vi "PTSequencer.execute step.vi"(0 "i ref in":refnum<vi>, 3 "ms timeout (10000)":i32=10000, 5 "error in (no error)":errorcluster) -> (14 "i ref out":refnum<vi>, 16 "next step":string, 17 "timed out":bool, 19 "error out":errorcluster)   [LabVIEW 2014, in "PTSequencer.lvlib"]
uses:
  PTSequencer.lvlib
  CS_Core/BaseProcess/BaseProcess.lvlib
  CS_Core/CSSystem/CSSystemLib/CSSystemLib.lvlib
  CS_Core/BaseSM/BaseSM.lvlib
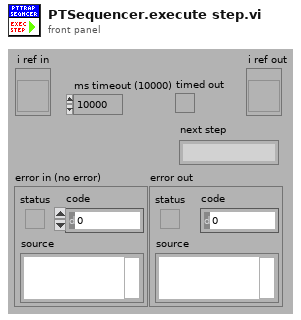
[diagram p1: front panel]
types:
  T1 = typedef "PTSequencer.lvlib/PTSequencer.i attribute.ctl" = cluster{"subsequence":bool, "mode":T2, "i step":i32, "nofLoops":i32, "i loop":i32, "Running":bool, "Paused":bool, "step done":bool, "loop done":bool, "seq done":bool, "DIM IDs":cluster{"step done":i32, "loop done":i32, "seq done":i32, "i step":i32, "i loop":i32}, "use stop conditions":bool, "stop conditions":T3[], "Step List":T5[], "DIM subsriptions":string[], "stop cond indexes":i32[], "step cond indexes":cluster{"step condition IDs":cluster{"step ID":i32, "condition ID":i32}[]}[], "Delay Start Time":timestamp, "status":string, "stopping":bool}
  T2 = typedef "PTSequencer.lvlib/PTSequencer.mode.ctl" = enum16{"single", "loop", "for loop"}
  T3 = typedef "PTSequencer.lvlib/PTSequencer.DIM service condition.ctl" = cluster{"DIM service":string, "descr":string, "nomValue":T4, "actValue":T4, "matched":bool, "DIM Status":cluster{"no link":bool, "quality":i32, "Time Stamp":timestamp}}
  T4 = typedef "CoreDefs.rawDataType.ctl" = i8[]
  T5 = typedef "PTSequencer.lvlib/PTSequencer.step.ctl" = cluster{"description":string, "object parameters":cluster{"object":string, "selector":string, "descriptor":string, "data":T4, "subsequence":bool, "call mode":enum16{"Simple DIM", "Synchronous"}, "data in":T4}, "result action":cluster{"check":bool, "passed":enum16{"Next", "Previous", "Repeat", "Jump"}, "failed":enum16{"Next", "Previous", "Repeat", "Jump"}, "jumpID_passed":i32, "jumpID_failed":i32}, "conditions":T3[], "fulfilled ":bool, "use delay":bool, "delay time (s)":dbl, "ID":i32}
  T6 = typedef "CoreDefs.call_type.ctl" = cluster{"Object":string, "Selector":string, "CallType":enum16{"simple", "synchronous", "asynchronous"}, "Async Object":string, "Async Selector":string, "Data Descriptor":T7, "Data":T4, "Error #":i32, "Expire":u32}
  T7 = typedef "BaseProcess.lvlib/BaseProcess.descriptor string definition.ctl" = string
  T8 = typedef "BaseSM.lvlib/BaseSM.i attribute.ctl" = cluster{"stateError":i32, "stateStatus":string, "stateQuality":T9, "ProcStateRef":refnum<vi>, "thread ref":refnum<vi>, "actState":string, "reqState":string, "SMQueue":refnum<queue>, "stateErrorID":i32, "stateStatusID":i32}
  T9 = typedef "BaseSM.lvlib/BaseSM.stateQuality.ctl" = i16
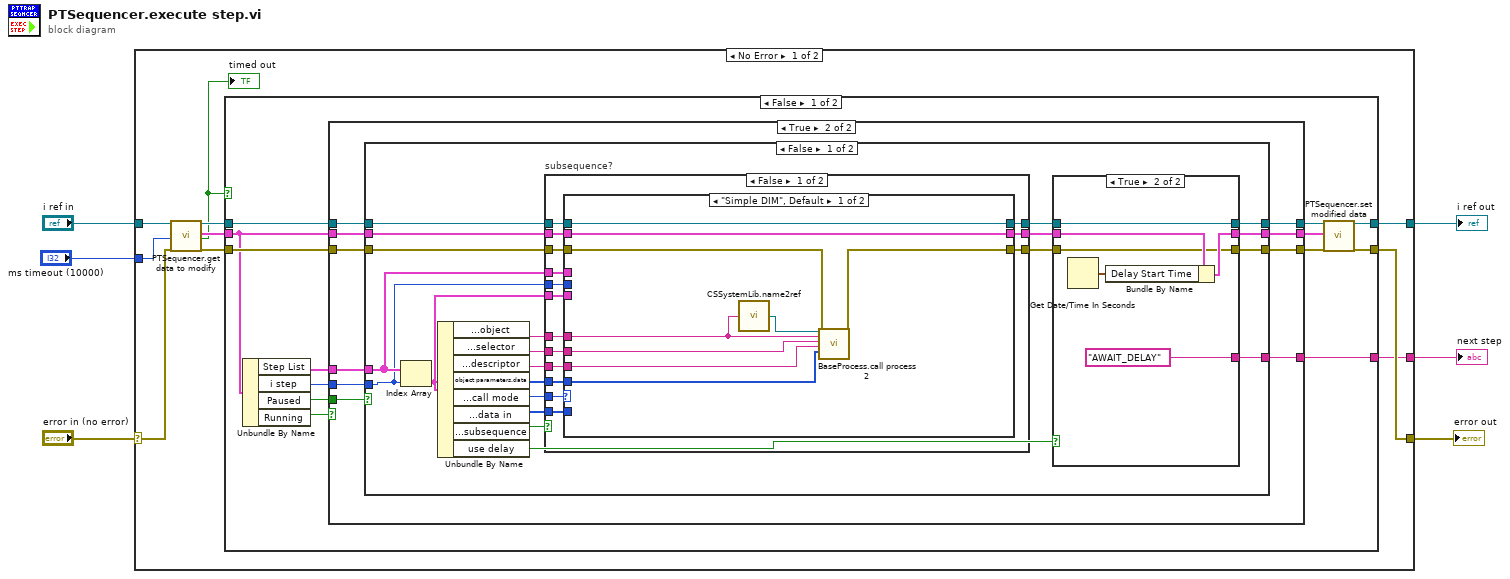
[diagram p0: block diagram]
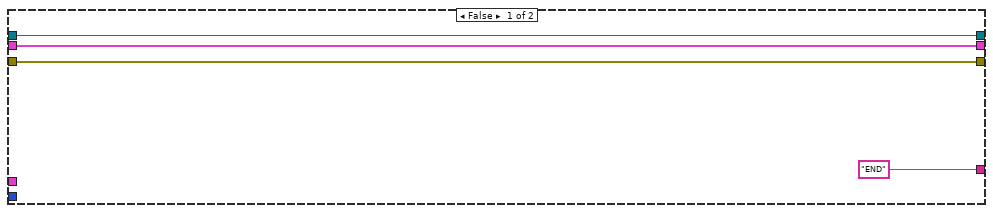
[diagram p2: hidden frame]
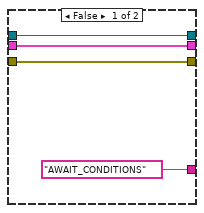
[diagram p3: hidden frame]
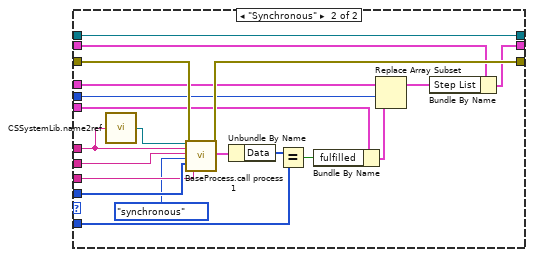
[diagram p4: hidden frame]
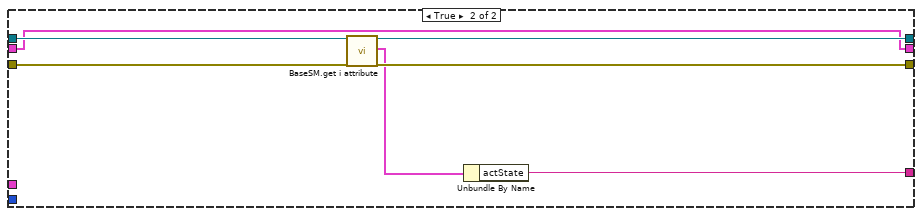
[diagram p6: hidden frame]
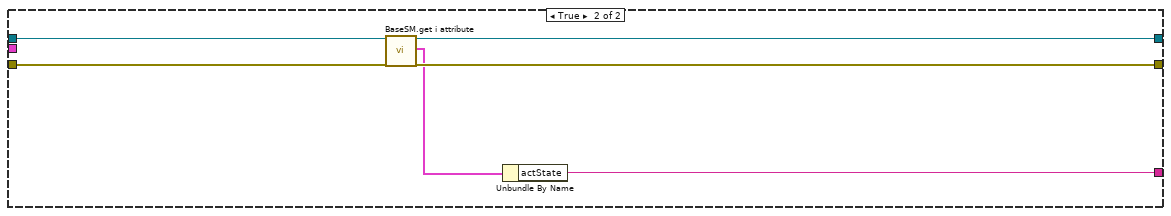
[diagram p7: hidden frame]
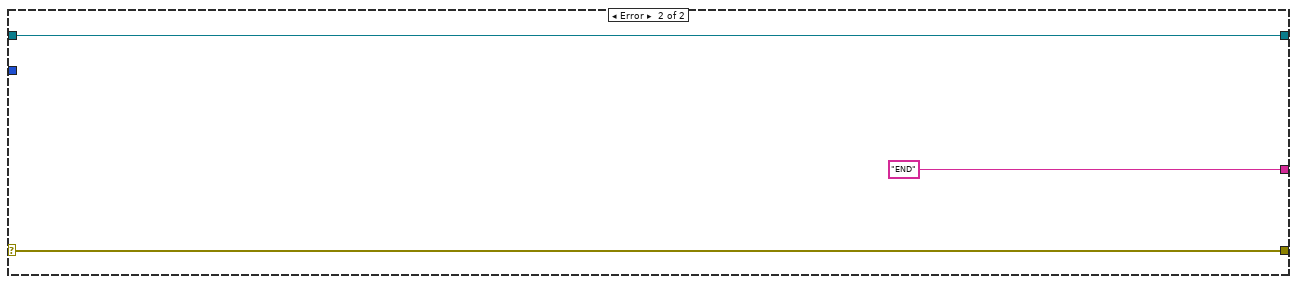
[diagram p8: hidden frame]
diagram:
  n1 = case shown="No Error" "error in (no error)" {
    selector: "error in (no error)" -> [w12 w136]
    tunnel: "i ref in" -> [w16 w137]
    tunnel: [w10 w136] -> w5
    tunnel: [w11 w137] -> w4
    tunnel: "ms timeout (10000)" -> [w8 _]
    tunnel: [w7 "END"] -> w1
    frame No Error {
      n2 = call "PTSequencer.get data to modify.vi"("i ref in"=w16, "ms timeout (10000)"=w8, "error in (no error)"=w12) -> ("i ref out"=w13:refnum<vi>, "i attribute"=w15:T1, "timed out"=w9:bool, "error out"=w14:errorcluster)  [unwired: 13 in]
      "timed out" <- w9
      n3 = case shown="False" w9 {
        tunnel: w15 -> [w23 _]
        tunnel: w14 -> [w29 w133]
        tunnel: w13 -> [w28 w134]
        tunnel: [w27 w132] -> w11
        tunnel: [w25 w131] -> w10
        tunnel: [w19 w129] -> w7
        frame False {
          n4 = Unbundle By Name(w23) -> ("Step List"=w22:T5[], "i step"=w21:i32, "Paused"=w17:bool, "Running"=w18:bool)
          n5 = case shown="True" w18 {
            tunnel: w29 -> [w30 w43]
            tunnel: w28 -> [w32 w42]
            tunnel: [w32 w41] -> w26
            tunnel: [w30 w40] -> w24
            tunnel: w23 -> [w31 w39]
            tunnel: w22 -> [_ w38]
            tunnel: w21 -> [_ w37]
            tunnel: [w31 w36] -> w20
            tunnel: ["END" w35] -> w19
            tunnel: w17 -> [_ w34]
            frame False {
            }
            frame True {
              n6 = case shown="False" w34 {
                tunnel: w43 -> [w63 w127]
                tunnel: w42 -> [w62 w128]
                tunnel: [w46 w126] -> w41
                tunnel: [w44 w125] -> w40
                tunnel: w39 -> [w57 w122]
                tunnel: w38 -> [w54 _]
                tunnel: w37 -> [w53 _]
                tunnel: [w49 w122] -> w36
                tunnel: [w48 w123] -> w35
                frame False {
                  n7 = Index Array(array=w54, index=w53) -> (element=w52:T5)
                  n8 = Unbundle By Name(w52) -> ("object parameters.object"=w61:string, "object parameters.selector"=w60:string, "object parameters.descriptor"=w59:string, "object parameters.data"=w58:T4, "object parameters.call mode"=w56:enum16{"Simple DIM", "Synchronous"}, "object parameters.data in"=w55:T4, "object parameters.subsequence"=w64:bool, "use delay"=w51:bool)
                  n9 = case "subsequence?" shown="False" w64 {
                    tunnel: w63 -> [w85 w119]
                    tunnel: w62 -> [w80 w121]
                    tunnel: w61 -> [w89 _]
                    tunnel: w60 -> [w88 _]
                    tunnel: w59 -> [w87 _]
                    tunnel: w58 -> [w86 _]
                    tunnel: [w79 w121] -> w47
                    tunnel: [w84 w119] -> w45
                    tunnel: [w78 w120] -> w50
                    tunnel: w57 -> [w81 w120]
                    tunnel: w56 -> [w83 _]
                    tunnel: w55 -> [w82 _]
                    tunnel: w54 -> [w77 _]
                    tunnel: w53 -> [w76 _]
                    tunnel: w52 -> [w75 _]
                    frame False {
                      n10 = case shown="\"Simple DIM\", Default" w83 {
                        tunnel: w89 -> [w97 w117]
                        tunnel: w88 -> [w96 w116]
                        tunnel: w87 -> [w95 w112]
                        tunnel: w86 -> [w90 w115]
                        tunnel: w85 -> [w94 w114]
                        tunnel: [w93 w113] -> w84
                        tunnel: w82 -> [_ w108]
                        tunnel: w81 -> [w91 w107]
                        tunnel: w80 -> [w92 w102]
                        tunnel: [w92 w102] -> w79
                        tunnel: [w91 w103] -> w78
                        tunnel: w77 -> [_ w106]
                        tunnel: w76 -> [_ w104]
                        tunnel: w75 -> [_ w101]
                        frame "Simple DIM", Default {
                          n11 = call "CSSystemLib.name2ref.vi"("name"=w97) -> ("obj refnum"=w98:refnum<vi>)
                          n12 = call "BaseProcess.call process 2.vi"("i ref in"=w98, "Object"=w97, "Selector"=w96, "Data Descriptor"=w95, "Data"=w90, "error in (no error)"=w94) -> ("error out"=w93:errorcluster)  [unwired: 12 in, 1 out]
                        }
                        frame "Synchronous" {
                          n13 = call "CSSystemLib.name2ref.vi"("name"=w117) -> ("obj refnum"=w118:refnum<vi>)
                          n14 = call "BaseProcess.call process 1.vi"("i ref in"=w118, "Object"=w117, "Selector"=w116, "CallType"=enum16{"simple", "synchronous", "asynchronous"}."synchronous", "Data"=w115, "error in (no error)"=w114, "Data Descriptor"=w112) -> ("call cluster out"=w110:T6, "error out"=w113:errorcluster)  [unwired: 10 in, 1 out]
                          n15 = Unbundle By Name(w110) -> ("Data"=w109:T4)
                          n16 = Equal?(x=w109, y=w108) -> (x = y?=w100:bool)
                          n17 = Bundle By Name(cluster=w101, "fulfilled"=w100) -> (w99:T5)
                          n18 = Replace Array Subset(array=w106, new element=w99, index=w104) -> (w105:T5[])
                          n19 = Bundle By Name(cluster=w107, "Step List"=w105) -> (w103:T1)
                        }
                      }
                    }
                    frame True {
                    }
                  }
                  n20 = case shown="True" w51 {
                    tunnel: w50 -> [w68 w74]
                    tunnel: [w68 w72] -> w49
                    tunnel: ["AWAIT_CONDITIONS" "AWAIT_DELAY"] -> w48
                    tunnel: w47 -> [w66 w70]
                    tunnel: [w66 w70] -> w46
                    tunnel: w45 -> [w65 w69]
                    tunnel: [w65 w69] -> w44
                    frame False {
                    }
                    frame True {
                      n21 = Get Date/Time In Seconds() -> (seconds since 1Jan1904=w73:timestamp)
                      n22 = Bundle By Name(cluster=w74, "Delay Start Time"=w73) -> (w72:T1)
                    }
                  }
                }
                frame True {
                  n23 = call "BaseSM.get i attribute.vi"("i ref in"=w128, "error in (no error)"=w127) -> ("i ref out"=w126:refnum<vi>, "i attribute"=w124:T8, "error out"=w125:errorcluster)  [unwired: 15 in]
                  n24 = Unbundle By Name(w124) -> ("actState"=w123:string)
                }
              }
            }
          }
          n25 = call "PTSequencer.set modified data.vi"("i ref in"=w26, "CLASS.i attribute"=w20, "error in (no error)"=w24) -> ("i ref out"=w27:refnum<vi>, "error out"=w25:errorcluster)  [unwired: 15 in]
        }
        frame True {
          n26 = call "BaseSM.get i attribute.vi"("i ref in"=w134, "error in (no error)"=w133) -> ("i ref out"=w132:refnum<vi>, "i attribute"=w130:T8, "error out"=w131:errorcluster)  [unwired: 15 in]
          n27 = Unbundle By Name(w130) -> ("actState"=w129:string)
        }
      }
    }
    frame Error {
    }
  }
  "error out" <- w5
  "i ref out" <- w4
  "next step" <- w1
